vi "Read Value (Type Code).vi"(7 "field name":string, 8 "error in (no error)":errorcluster, 9 "type code":T1, 10 "value":variant, 11 "Value in":refnum<class "Value.lvclass">) -> (0 "error out":errorcluster, 2 "value out":variant, 3 "Value out":refnum<class "Value.lvclass">)   [LabVIEW 2020, in "Value.lvlib" / "Value.lvclass"]
uses:
  Value.lvclass
  Value.lvclass/Value.ctl
  <vilib>/ErrorRing/Error Ring.xnode
  3e63842f-1b42-44b7-bfbc-53574ae558bd.vi
  0df52538-0c37-4fc1-a2a6-aa64d23bd73e.vi
  ea7cb730-9445-4e63-a674-7488b051f0a2.vi
  ecc6d044-d1d6-4258-b554-93b542f000c4.vi
  f0dd0353-13dc-4229-be36-72f5216b3ba3.vi
  663b7534-5be4-4c26-8693-775dffd107bf.vi
  6d95b702-a3d4-47fa-b99c-6e9c691d9abd.vi
  334379f0-c2c1-4fd4-b37a-a75153a3c3c1.vi
  22215a59-2fe5-468e-8a76-07a567f1422d.vi
  3b673ad6-c2bb-415d-ac32-dac8d0585a62.vi
  4907590c-51dd-452d-854a-3f23d6337043.vi
  91e94b60-106e-4a8f-bb72-5d9817169e6a.vi
  c7390ac7-e1e0-4f30-b90a-9159575d946d.vi
  aaf6655d-cd8e-45f8-b77e-a22837ed21e0.vi
  830d96f2-0dcb-4e12-99cb-9e6dde05f73e.vi
  77dc8c9c-6059-4e17-8748-14fb7ec0ac2f.vi
  a9875d30-4bd9-4a8c-a52c-f68dec12aa6b.vi
  6dbc08b8-92b8-4054-99f1-d97896c52856.vi
  c55a9e90-05cb-4a8a-8098-6274f5663967.vi
  316c9c8d-b543-4ebf-942d-59175514938d.vi
  229b0493-3b28-4ef3-8240-f1556a969e00.vi
  76e9d66a-8186-463b-a0b5-702645c41f9e.vi
  c324c6c0-264f-44f1-9003-e2f03347ce10.vi
  99229403-bf4d-41b1-8e34-2119cf99b534.vi
  94649a53-8ca4-4095-9f16-4726c07ca332.vi
  d57c28cb-9096-4c65-b10b-a5dea6344eea.vi
  a983453c-48a8-483e-9635-4b6015360bbf.vi
  3184ba56-7df3-4453-b731-c59013ebea68.vi
  6054442b-7a6b-42bc-83b9-383781339b04.vi
  6affac03-527b-4ec4-b0fc-9a513264455a.vi
  a9131e02-a07e-4dd8-b605-98a98183cd4d.vi
  df721e5c-d840-4c3d-88a1-754951405b27.vi
  37bd5290-b6b7-48eb-a0fa-e2d498b26fe2.vi
  1f354738-e960-4e7d-8bfb-2b975031cf57.vi
  eb45627c-0224-4171-a2ca-7d038fcf7cb5.vi
  763b9c78-21ee-42ab-85a7-a612ad3e0854.vi
  b475763c-3eeb-44d5-9789-6e92f77c8c05.vi
  7e13b756-e5dd-4f30-8145-3e48ab5751a0.vi
  311b836b-25cf-44d6-867a-da423852ab29.vi
  884a57a7-1cc5-4241-a283-3421418f3c32.vi
  e5b34253-12a8-4f36-ae48-ef8a9a19dc9f.vi
  9a6462e7-f1a7-4896-b94c-43e163632ccd.vi
  919939b4-f74b-49d6-a078-a721f5adc92b.vi
  7b5734c8-9551-4087-a43c-2e9c6be36d77.vi
  e7c0ed72-c8d2-4a6e-8d95-57b650344be6.vi
  78a636ab-c8c7-43d5-9c2f-ed25fd418a22.vi
  3f976d8e-f489-4d6c-8102-c644feb36fb3.vi
  2b071918-53f3-414b-a359-069b1376627a.vi
  <vilib>/Utility/error.llb/Error Cluster From Error Code.vi
  Type Code.ctl
  Value.lvlib
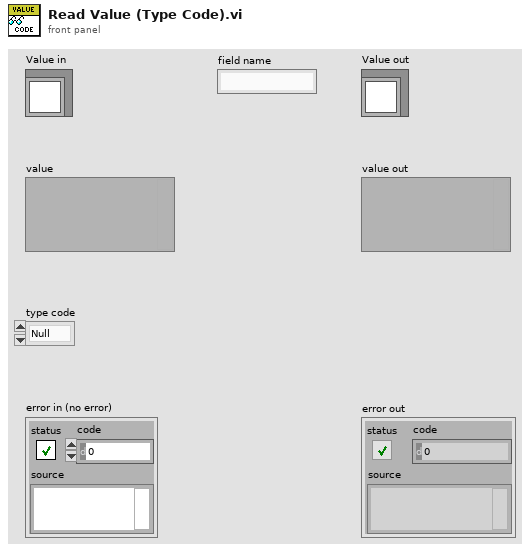
[diagram p1: front panel]
types:
  T1 = typedef "Value.lvlib/Type Code.ctl" = enum8{"Null", "Bool", "BoolA", "Int8", "Int8A", "Int16", "Int16A", "Int32", "Int32A", "Int64", "Int64A", "UInt8", "UInt8A", "UInt16", "UInt16A", "UInt32", "UInt32A", "UInt64", "UInt64A", "Float32", "Float32A", "Float64", "Float64A", "String", "StringA", "Struct", "StructA", "Union", "UnionA", "Any", "AnyA"}
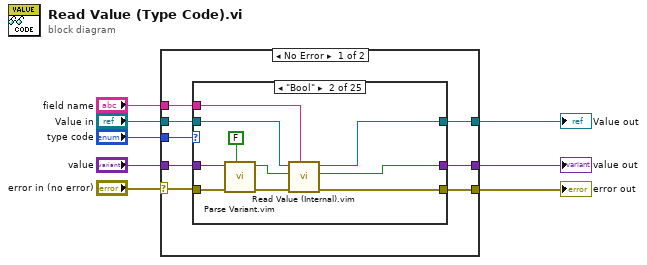
[diagram p0: block diagram]
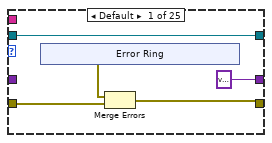
[diagram p2: hidden frame]
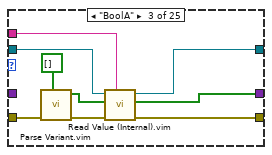
[diagram p3: hidden frame]
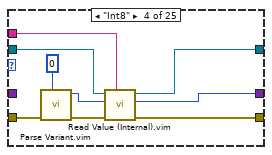
[diagram p4: hidden frame]
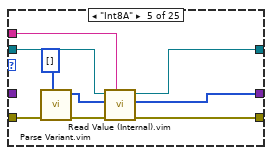
[diagram p5: hidden frame]
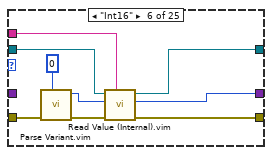
[diagram p6: hidden frame]
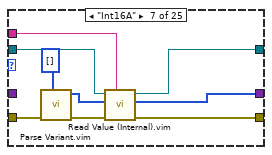
[diagram p7: hidden frame]
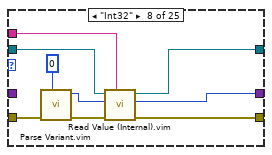
[diagram p8: hidden frame]
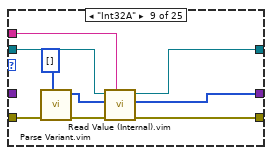
[diagram p9: hidden frame]
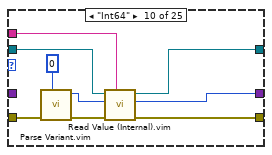
[diagram p10: hidden frame]
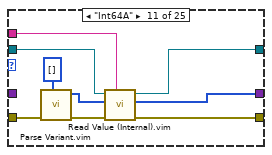
[diagram p11: hidden frame]
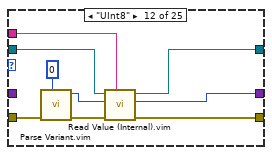
[diagram p12: hidden frame]
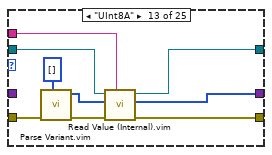
[diagram p13: hidden frame]
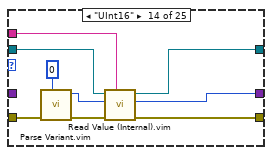
[diagram p14: hidden frame]
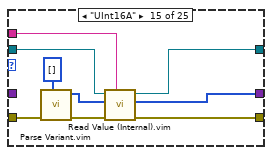
[diagram p15: hidden frame]
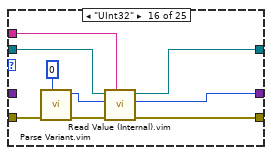
[diagram p16: hidden frame]
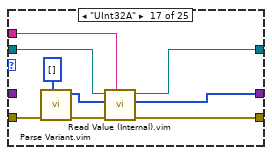
[diagram p17: hidden frame]
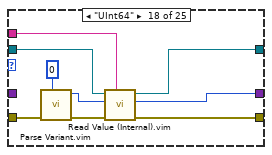
[diagram p18: hidden frame]
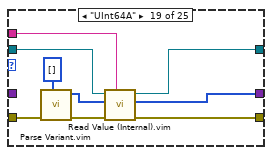
[diagram p19: hidden frame]
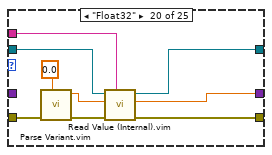
[diagram p20: hidden frame]
diagram:
  n1 = case shown="No Error" "error in (no error)" {
    selector: "error in (no error)" -> [w11 w245]
    tunnel: [w16 w243] -> w7
    tunnel: [w15 w245] -> w6
    tunnel: "Value in" -> [w14 w244]
    tunnel: [w13 w244] -> w4
    tunnel: "field name" -> [w12 _]
    tunnel: "value" -> [w10 w243]
    tunnel: "type code" -> [w9 _]
    frame No Error {
      n2 = case shown="\"Bool\"" w9 {
        tunnel: [w20 w32 w42 w51 w60 w69 w78 w87 w96 w105 w115 w123 w132 w141 w150 w159 w168 w177 w186 w195 w204 w213 w222 w231 w240] -> w15
        tunnel: w11 -> [w21 w35 w44 w53 w62 w71 w80 w89 w98 w107 w116 w125 w134 w143 w152 w161 w170 w179 w188 w197 w206 w215 w224 w233 w242]
        tunnel: [w17 w30 w40 w50 w58 w67 w76 w85 w94 w103 w113 w121 w130 w140 w148 w157 w167 w175 w184 w193 w202 w211 w220 w229 w238] -> w13
        tunnel: [variant w29 w38 w48 w56 w65 w74 w83 w92 w101 w111 w119 w128 w138 w146 w155 w165 w173 w182 w191 w200 w209 w218 w227 w236] -> w16
        tunnel: w14 -> [w17 w28 w37 w47 w55 w64 w73 w82 w91 w100 w109 w118 w127 w137 w145 w154 w164 w172 w181 w190 w199 w208 w217 w226 w235]
        tunnel: w12 -> [_ w27 w36 w45 w54 w63 w72 w81 w90 w99 w108 w117 w126 w135 w144 w153 w162 w171 w180 w189 w198 w207 w216 w225 w234]
        tunnel: w10 -> [_ w26 _ _ _ _ _ _ _ _ _ _ _ _ _ _ _ _ _ _ _ _ _ _ _]
        frame Default {
          n3 = xnode "Error Ring"() -> ("error out"=w19:errorcluster)
          n4 = Merge Errors(w19, w21) -> (w20:errorcluster)
        }
        frame "Bool" {
          n5 = call "Parse Variant.vim"("default"=FALSE, "error in (no error)"=w35, "value"=w26) -> ("error out"=w33:errorcluster, "value out"=w31:bool)  [unwired: 7 in]
          n6 = call "Read Value (Internal).vim"("field name"=w27, "error in"=w33, "default"=w31, "Value in"=w28) -> ("error out"=w32:errorcluster, "value"=w29:bool, "Value out"=w30:refnum<class "Value.lvclass">)  [unwired: 5 in]
        }
        frame "BoolA" {
          n7 = call "Parse Variant.vim"("default"=bool[] [], "error in (no error)"=w44) -> ("error out"=w43:errorcluster, "value out"=w41:bool[])  [unwired: 8 in]
          n8 = call "Read Value (Internal).vim"("field name"=w36, "error in"=w43, "default"=w41, "Value in"=w37) -> ("error out"=w42:errorcluster, "value"=w38:bool[], "Value out"=w40:refnum<class "Value.lvclass">)  [unwired: 5 in]
        }
        frame "Int8" {
          n9 = call "Parse Variant.vim"("default"=i8 0, "error in (no error)"=w53) -> ("error out"=w52:errorcluster, "value out"=w46:i8)  [unwired: 8 in]
          n10 = call "Read Value (Internal).vim"("field name"=w45, "error in"=w52, "default"=w46, "Value in"=w47) -> ("error out"=w51:errorcluster, "value"=w48:i8, "Value out"=w50:refnum<class "Value.lvclass">)  [unwired: 5 in]
        }
        frame "Int8A" {
          n11 = call "Parse Variant.vim"("default"=i8[] [], "error in (no error)"=w62) -> ("error out"=w61:errorcluster, "value out"=w59:i8[])  [unwired: 8 in]
          n12 = call "Read Value (Internal).vim"("field name"=w54, "error in"=w61, "default"=w59, "Value in"=w55) -> ("error out"=w60:errorcluster, "value"=w56:i8[], "Value out"=w58:refnum<class "Value.lvclass">)  [unwired: 5 in]
        }
        frame "Int16" {
          n13 = call "Parse Variant.vim"("default"=i16 0, "error in (no error)"=w71) -> ("error out"=w70:errorcluster, "value out"=w68:i16)  [unwired: 8 in]
          n14 = call "Read Value (Internal).vim"("field name"=w63, "error in"=w70, "default"=w68, "Value in"=w64) -> ("error out"=w69:errorcluster, "value"=w65:i16, "Value out"=w67:refnum<class "Value.lvclass">)  [unwired: 5 in]
        }
        frame "Int16A" {
          n15 = call "Parse Variant.vim"("default"=i16[] [], "error in (no error)"=w80) -> ("error out"=w79:errorcluster, "value out"=w77:i16[])  [unwired: 8 in]
          n16 = call "Read Value (Internal).vim"("field name"=w72, "error in"=w79, "default"=w77, "Value in"=w73) -> ("error out"=w78:errorcluster, "value"=w74:i16[], "Value out"=w76:refnum<class "Value.lvclass">)  [unwired: 5 in]
        }
        frame "Int32" {
          n17 = call "Parse Variant.vim"("default"=0, "error in (no error)"=w89) -> ("error out"=w88:errorcluster, "value out"=w86:i32)  [unwired: 8 in]
          n18 = call "Read Value (Internal).vim"("field name"=w81, "error in"=w88, "default"=w86, "Value in"=w82) -> ("error out"=w87:errorcluster, "value"=w83:i32, "Value out"=w85:refnum<class "Value.lvclass">)  [unwired: 5 in]
        }
        frame "Int32A" {
          n19 = call "Parse Variant.vim"("default"=i32[] [], "error in (no error)"=w98) -> ("error out"=w97:errorcluster, "value out"=w95:i32[])  [unwired: 8 in]
          n20 = call "Read Value (Internal).vim"("field name"=w90, "error in"=w97, "default"=w95, "Value in"=w91) -> ("error out"=w96:errorcluster, "value"=w92:i32[], "Value out"=w94:refnum<class "Value.lvclass">)  [unwired: 5 in]
        }
        frame "Int64" {
          n21 = call "Parse Variant.vim"("default"=i64 0, "error in (no error)"=w107) -> ("error out"=w106:errorcluster, "value out"=w104:i64)  [unwired: 8 in]
          n22 = call "Read Value (Internal).vim"("field name"=w99, "error in"=w106, "default"=w104, "Value in"=w100) -> ("error out"=w105:errorcluster, "value"=w101:i64, "Value out"=w103:refnum<class "Value.lvclass">)  [unwired: 5 in]
        }
        frame "Int64A" {
          n23 = call "Parse Variant.vim"("default"=i64[] [], "error in (no error)"=w116) -> ("error out"=w110:errorcluster, "value out"=w114:i64[])  [unwired: 8 in]
          n24 = call "Read Value (Internal).vim"("field name"=w108, "error in"=w110, "default"=w114, "Value in"=w109) -> ("error out"=w115:errorcluster, "value"=w111:i64[], "Value out"=w113:refnum<class "Value.lvclass">)  [unwired: 5 in]
        }
        frame "UInt8" {
          n25 = call "Parse Variant.vim"("default"=u8 0, "error in (no error)"=w125) -> ("error out"=w124:errorcluster, "value out"=w122:u8)  [unwired: 8 in]
          n26 = call "Read Value (Internal).vim"("field name"=w117, "error in"=w124, "default"=w122, "Value in"=w118) -> ("error out"=w123:errorcluster, "value"=w119:u8, "Value out"=w121:refnum<class "Value.lvclass">)  [unwired: 5 in]
        }
        frame "UInt8A" {
          n27 = call "Parse Variant.vim"("default"=u8[] [], "error in (no error)"=w134) -> ("error out"=w133:errorcluster, "value out"=w131:u8[])  [unwired: 8 in]
          n28 = call "Read Value (Internal).vim"("field name"=w126, "error in"=w133, "default"=w131, "Value in"=w127) -> ("error out"=w132:errorcluster, "value"=w128:u8[], "Value out"=w130:refnum<class "Value.lvclass">)  [unwired: 5 in]
        }
        frame "UInt16" {
          n29 = call "Parse Variant.vim"("default"=u16 0, "error in (no error)"=w143) -> ("error out"=w142:errorcluster, "value out"=w136:u16)  [unwired: 8 in]
          n30 = call "Read Value (Internal).vim"("field name"=w135, "error in"=w142, "default"=w136, "Value in"=w137) -> ("error out"=w141:errorcluster, "value"=w138:u16, "Value out"=w140:refnum<class "Value.lvclass">)  [unwired: 5 in]
        }
        frame "UInt16A" {
          n31 = call "Parse Variant.vim"("default"=u16[] [], "error in (no error)"=w152) -> ("error out"=w151:errorcluster, "value out"=w149:u16[])  [unwired: 8 in]
          n32 = call "Read Value (Internal).vim"("field name"=w144, "error in"=w151, "default"=w149, "Value in"=w145) -> ("error out"=w150:errorcluster, "value"=w146:u16[], "Value out"=w148:refnum<class "Value.lvclass">)  [unwired: 5 in]
        }
        frame "UInt32" {
          n33 = call "Parse Variant.vim"("default"=u32 0, "error in (no error)"=w161) -> ("error out"=w160:errorcluster, "value out"=w158:u32)  [unwired: 8 in]
          n34 = call "Read Value (Internal).vim"("field name"=w153, "error in"=w160, "default"=w158, "Value in"=w154) -> ("error out"=w159:errorcluster, "value"=w155:u32, "Value out"=w157:refnum<class "Value.lvclass">)  [unwired: 5 in]
        }
        frame "UInt32A" {
          n35 = call "Parse Variant.vim"("default"=u32[] [], "error in (no error)"=w170) -> ("error out"=w169:errorcluster, "value out"=w163:u32[])  [unwired: 8 in]
          n36 = call "Read Value (Internal).vim"("field name"=w162, "error in"=w169, "default"=w163, "Value in"=w164) -> ("error out"=w168:errorcluster, "value"=w165:u32[], "Value out"=w167:refnum<class "Value.lvclass">)  [unwired: 5 in]
        }
        frame "UInt64" {
          n37 = call "Parse Variant.vim"("default"=u64 0, "error in (no error)"=w179) -> ("error out"=w178:errorcluster, "value out"=w176:u64)  [unwired: 8 in]
          n38 = call "Read Value (Internal).vim"("field name"=w171, "error in"=w178, "default"=w176, "Value in"=w172) -> ("error out"=w177:errorcluster, "value"=w173:u64, "Value out"=w175:refnum<class "Value.lvclass">)  [unwired: 5 in]
        }
        frame "UInt64A" {
          n39 = call "Parse Variant.vim"("default"=u64[] [], "error in (no error)"=w188) -> ("error out"=w187:errorcluster, "value out"=w185:u64[])  [unwired: 8 in]
          n40 = call "Read Value (Internal).vim"("field name"=w180, "error in"=w187, "default"=w185, "Value in"=w181) -> ("error out"=w186:errorcluster, "value"=w182:u64[], "Value out"=w184:refnum<class "Value.lvclass">)  [unwired: 5 in]
        }
        frame "Float32" {
          n41 = call "Parse Variant.vim"("default"=sgl 0.0, "error in (no error)"=w197) -> ("error out"=w196:errorcluster, "value out"=w194:sgl)  [unwired: 8 in]
          n42 = call "Read Value (Internal).vim"("field name"=w189, "error in"=w196, "default"=w194, "Value in"=w190) -> ("error out"=w195:errorcluster, "value"=w191:sgl, "Value out"=w193:refnum<class "Value.lvclass">)  [unwired: 5 in]
        }
        frame "Float64" {
          n43 = call "Parse Variant.vim"("default"=0.0, "error in (no error)"=w206) -> ("error out"=w205:errorcluster, "value out"=w203:dbl)  [unwired: 8 in]
          n44 = call "Read Value (Internal).vim"("field name"=w198, "error in"=w205, "default"=w203, "Value in"=w199) -> ("error out"=w204:errorcluster, "value"=w200:dbl, "Value out"=w202:refnum<class "Value.lvclass">)  [unwired: 5 in]
        }
        frame "Float32A" {
          n45 = call "Parse Variant.vim"("default"=sgl[] [], "error in (no error)"=w215) -> ("error out"=w214:errorcluster, "value out"=w212:sgl[])  [unwired: 8 in]
          n46 = call "Read Value (Internal).vim"("field name"=w207, "error in"=w214, "default"=w212, "Value in"=w208) -> ("error out"=w213:errorcluster, "value"=w209:sgl[], "Value out"=w211:refnum<class "Value.lvclass">)  [unwired: 5 in]
        }
        frame "Float64A" {
          n47 = call "Parse Variant.vim"("default"=dbl[] [], "error in (no error)"=w224) -> ("error out"=w223:errorcluster, "value out"=w221:dbl[])  [unwired: 8 in]
          n48 = call "Read Value (Internal).vim"("field name"=w216, "error in"=w223, "default"=w221, "Value in"=w217) -> ("error out"=w222:errorcluster, "value"=w218:dbl[], "Value out"=w220:refnum<class "Value.lvclass">)  [unwired: 5 in]
        }
        frame "String" {
          n49 = call "Parse Variant.vim"("default"="", "error in (no error)"=w233) -> ("error out"=w232:errorcluster, "value out"=w230:string)  [unwired: 8 in]
          n50 = call "Read Value (Internal).vim"("field name"=w225, "error in"=w232, "default"=w230, "Value in"=w226) -> ("error out"=w231:errorcluster, "value"=w227:string, "Value out"=w229:refnum<class "Value.lvclass">)  [unwired: 5 in]
        }
        frame "StringA" {
          n51 = call "Parse Variant.vim"("default"=string[] [], "error in (no error)"=w242) -> ("error out"=w241:errorcluster, "value out"=w239:string[])  [unwired: 8 in]
          n52 = call "Read Value (Internal).vim"("field name"=w234, "error in"=w241, "default"=w239, "Value in"=w235) -> ("error out"=w240:errorcluster, "value"=w236:string[], "Value out"=w238:refnum<class "Value.lvclass">)  [unwired: 5 in]
        }
      }
    }
    frame Error {
    }
  }
  "value out" <- w7
  "error out" <- w6
  "Value out" <- w4
